vi "Main Page.vi"(8 "error in (no error)":errorcluster, 11 "Node Ptr":T1 format="%.0x") -> (0 "error out":errorcluster)   [LabVIEW 2013, in "PWM System Explorer.lvlib"]
uses:
  PWM System Explorer.lvlib
  <vilib>/NI Veristand/Custom Device API/Custom Device Item Ref.ctl
  NationalInstruments.VeriStand.SystemStorage
  Shared/Constants.vi
  <vilib>/NI Veristand/Custom Device API/Get Item Property (Variant).vi
  <vilib>/NI Veristand/Custom Device API/Set Item Property (Variant).vi
  <vilib>/NI Veristand/Custom Device API/Set Item Property (Double).vi
  <vilib>/NI Veristand/Custom Device Tools/Custom Device Utility Library/NI VeriStand - Search for Item by Name.vi
  <vilib>/NI Veristand/Custom Device API/Custom Device API.lvlib
  <vilib>/NI Veristand/Custom Device Tools/Custom Device Utility Library/Custom Device Utility Library.lvlib
  Shared/PWM Shared.lvlib
panel:
  in  "Remove":bool
  in  "Add":bool
  in  "PWM channels in bitfile":i32[](listbox)=[3]
  in  "Header":cluster{"Section Name":string}={"Section Name"="Custom Device Item Settings"}
  in  "Description":string
  in  "Name":string
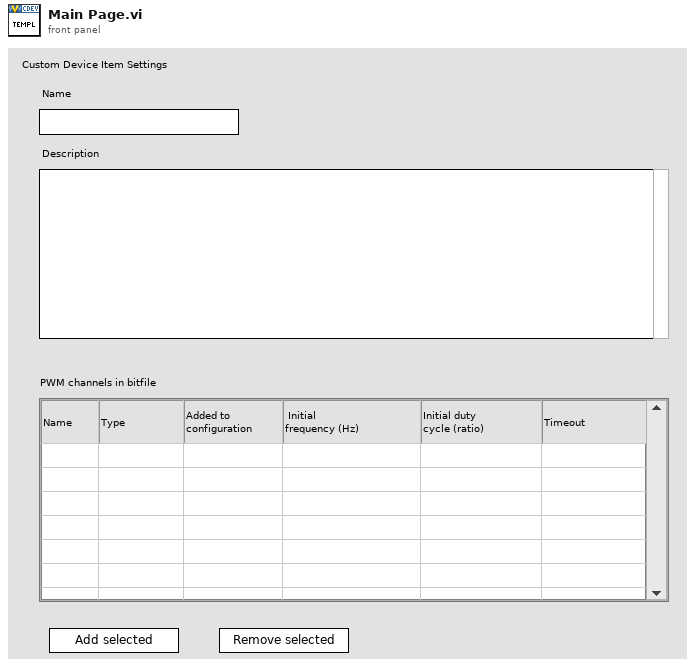
[diagram p1: front panel]
types:
  T1 = typedef "Custom Device API.lvlib/Custom Device Item Ref.ctl" = u64
  T2 = typedef "Custom Device API.lvlib/Custom Device Item Info.ctl" = cluster{"Name":string, "Is Channel":bool, "GUID":string, "Is Waveform":bool}
  T3 = typedef "Custom Device API.lvlib/Custom Device Commands.ctl" = enum16{"Default", "Item renamed", "Shutdown", "Dynamic button pressed"}
  T4 = typedef "Custom Device API.lvlib/Custom Device Pointer.ctl" = refnum<k24>
  T5 = typedef "LVPoint32TypeDef.ctl" = cluster{"Horizontal":i32, "Vertical":i32}
  T6 = typedef "LVRowAndColumnTypeDef.ctl" = cluster{"Row":i32, "Column":i32}
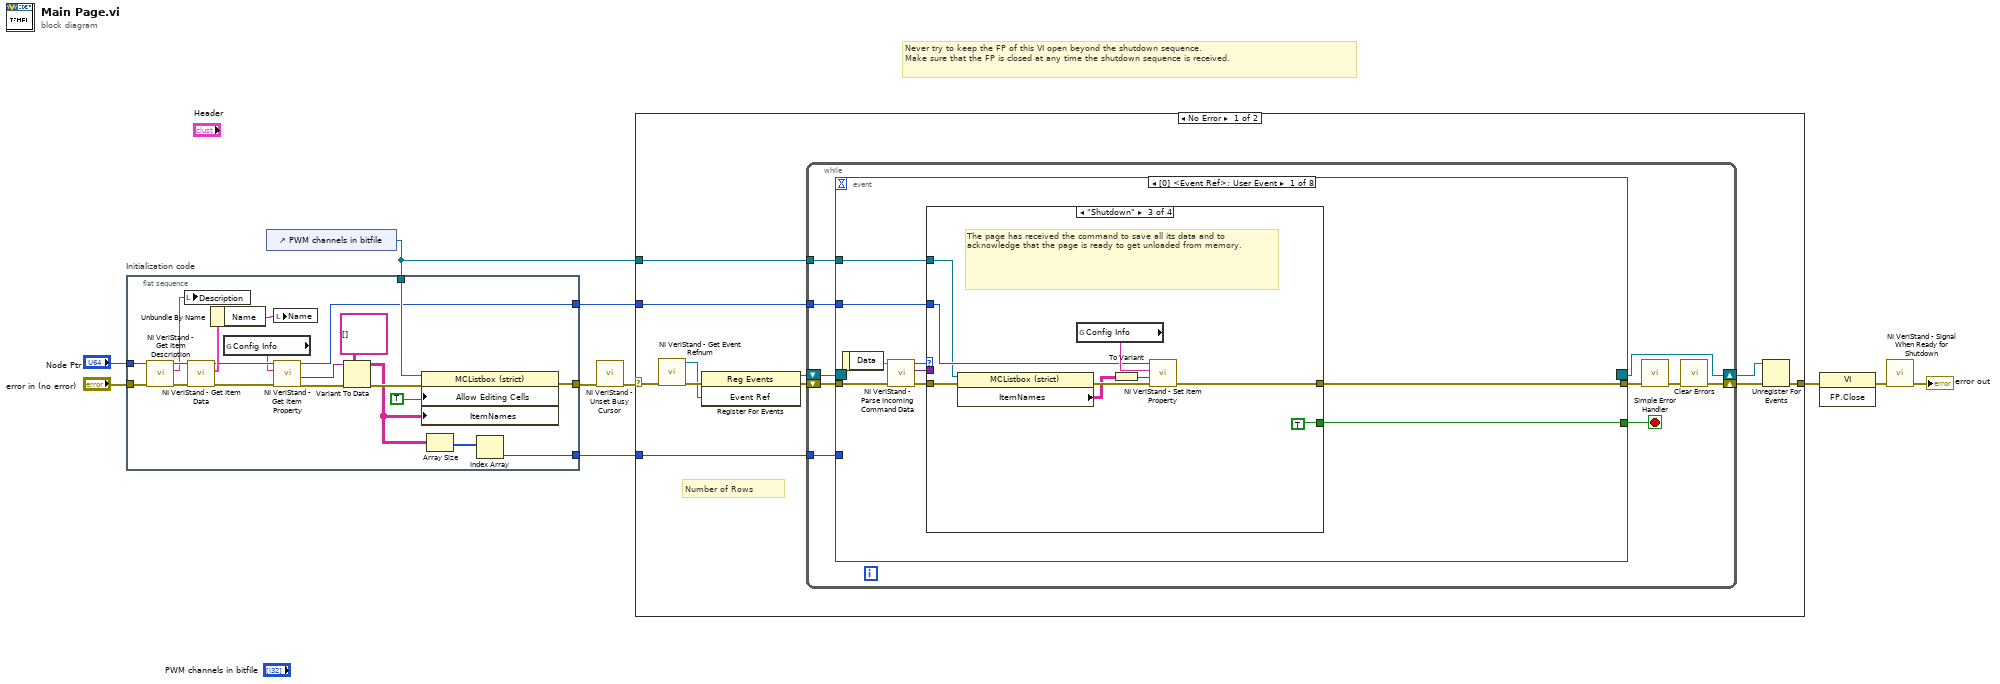
[diagram p0: block diagram]
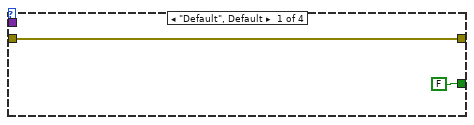
[diagram p2: hidden frame]
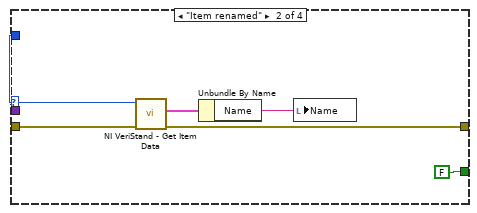
[diagram p3: hidden frame]
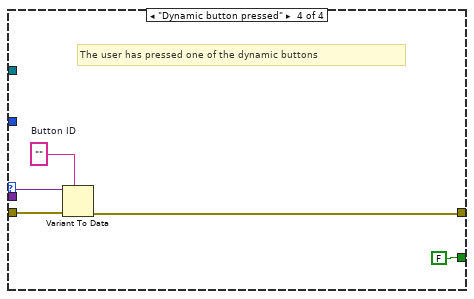
[diagram p4: hidden frame]
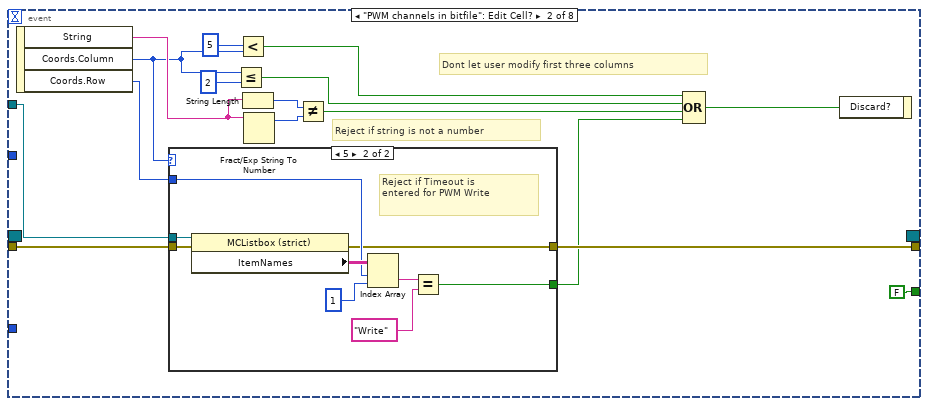
[diagram p5: hidden frame]
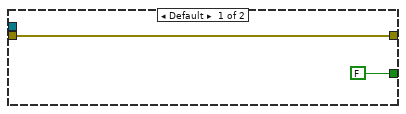
[diagram p6: hidden frame]
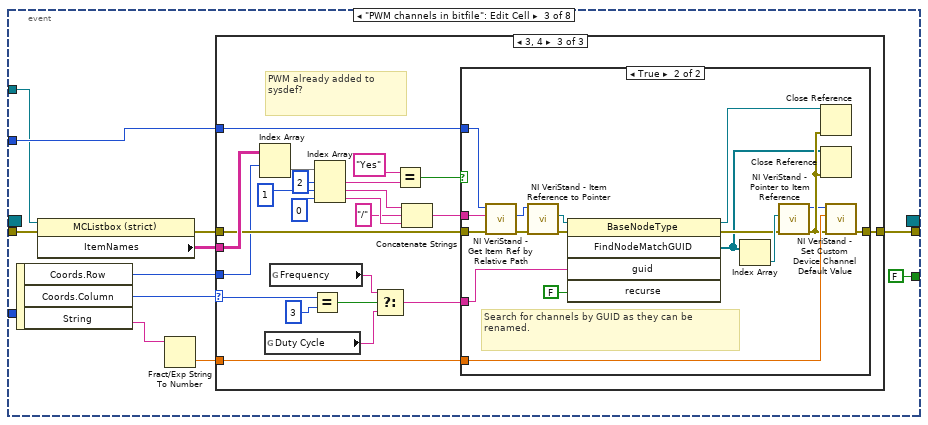
[diagram p7: hidden frame]
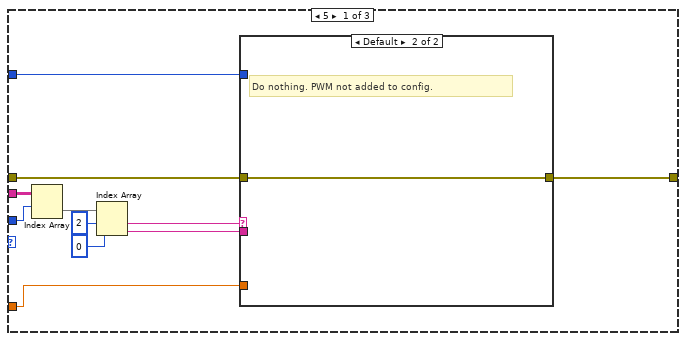
[diagram p8: hidden frame]
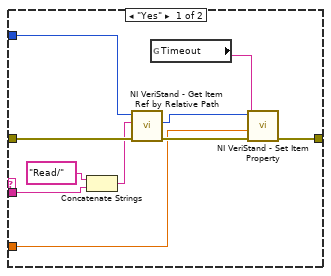
[diagram p9: hidden frame]
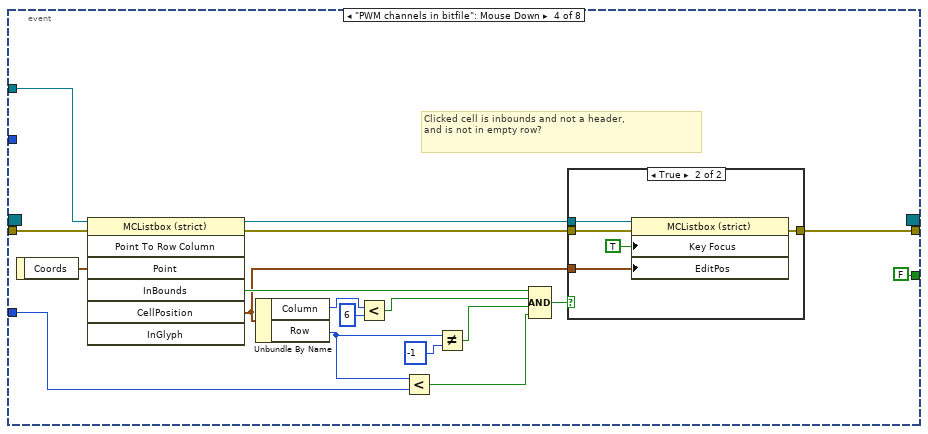
[diagram p12: hidden frame]
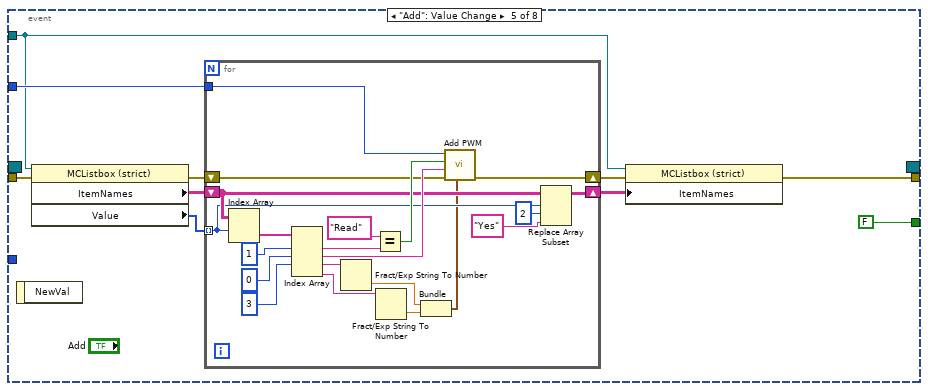
[diagram p14: hidden frame]
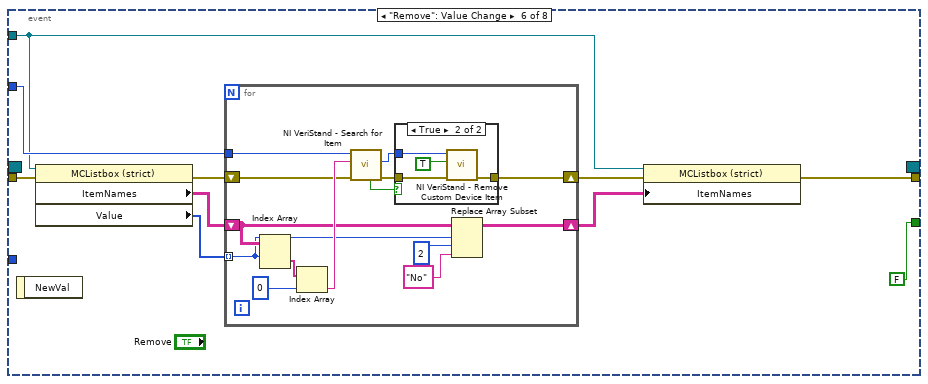
[diagram p15: hidden frame]
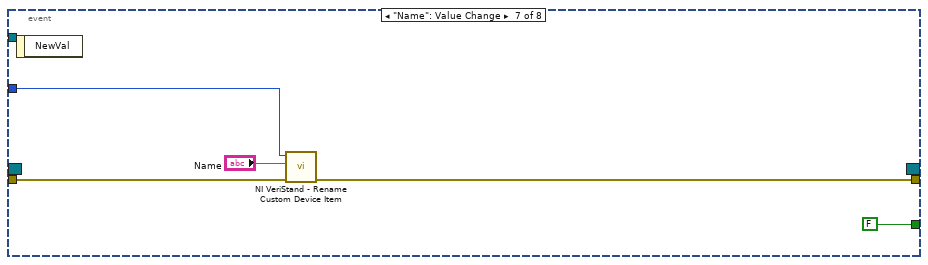
[diagram p17: hidden frame]
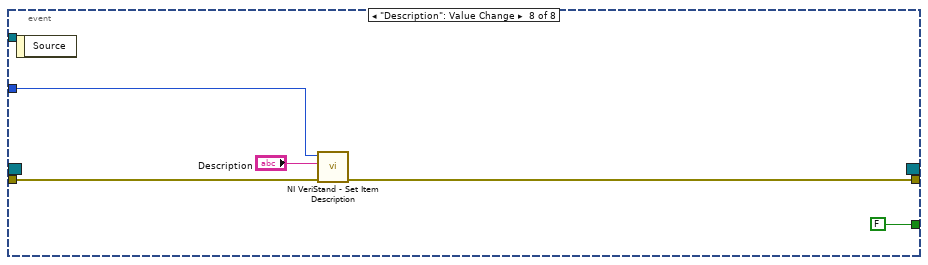
[diagram p18: hidden frame]
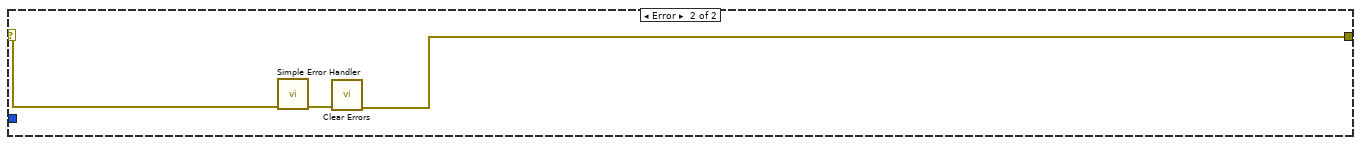
[diagram p19: hidden frame]
diagram:
  # "Never try to keep the FP of this VI open beyond the shutdown sequence.\nMake sure that the FP is closed at any time the shutdown sequence is received."
  n1 = flat-sequence "Initialization code" {
    tunnel: "error in (no error)" -> [w30]
    tunnel: "Node Ptr" -> [w29]
    tunnel: [w23] -> w6
    tunnel: [w17] -> w3
    tunnel: w2 -> [w24]
    tunnel: [w20] -> w1
    frame #0 {
      n2 = call <vilib>:"NI VeriStand - Get Item Description.vi"("error in (no error)"=w30, "Item Ref in"=w29) -> ("error out"=w27:errorcluster, "Description"=w28:string, "Item Ref out"=w31:T1)  [unwired: 7 out]
      n3 = local write "Description"(w28) -> ()
      n4 = call <vilib>:"NI VeriStand - Get Item Data.vi"("error in (no error)"=w27, "Item Ref in"=w31) -> ("error out"=w18:errorcluster, "Item Info"=w26:T2, "Item Ref out"=w19:T1)  [unwired: 7 out]
      n5 = Unbundle By Name(w26) -> ("Name"=w25:string)
      n6 = global read "Constants.vi" "Config Info"() -> (w11:string)
      n7 = local write "Name"(w25) -> ()
      n8 = call-poly <vilib>:"NI VeriStand - Get Item Property.vi"("error in (no error)"=w18, "Property Name"=w11, "Item Ref in"=w19) -> ("error out"=w14:errorcluster, "Value"=w15:variant, "Item Ref out"=w17:T1)  [unwired: 5 in, 1 out]
      n9 = Variant To Data(error in=w14, type=string[][] [] ("Item Names"), Variant=w15) -> (data=w12:string[][], error out=w13:errorcluster)
      n10 = property class="MCListbox (strict)"(reference=w24, error in=w13, "Allow Editing Cells"=TRUE, "ItemNames"=w12) -> (error out=w23:errorcluster)  [unwired: 1 out]
      n11 = Array Size(array=w12) -> (size(s)=w21:i32[])
      n12 = Index Array(array=w21) -> (element=w20:i32)  [unwired: 1 in]
    }
  }
  n13 = control-ref of="PWM channels in bitfile"() -> (w2:refnum<vi>)
  n14 = call <vilib>:"NI VeriStand - Unset Busy Cursor.vi"("error in (no error)"=w6) -> ("error out"=w5:errorcluster)  [unwired: 10 out]
  n15 = case shown="No Error" w5 {
    selector: w5 -> [w35 w282]
    tunnel: [w39 w280] -> w10
    tunnel: w3 -> [w34 _]
    tunnel: w2 -> [w33 _]
    tunnel: w1 -> [w32 _]
    frame No Error {
      # "Number of Rows"
      n16 = call <vilib>:"NI VeriStand - Get Event Refnum.vi"("error in (no error)"=w35) -> ("error out"=w42:errorcluster, "Event Ref"=w38:refnum<user-event>)  [unwired: 9 out]
      n17 = register-events(error in=w42, w38) -> (reference out=w36:refnum<event-registration>, error out=w37:errorcluster)  [unwired: 1 in]
      n18 = while {
        tunnel: w34 -> [w48]
        shift-right: [w45] -> w40
        shift-left: w37 -> [w51]
        shift-right: [w52] -> w41
        shift-left: w36 -> [w50]
        tunnel: w33 -> [w44]
        tunnel: w32 -> [w43]
        stop <- w49 stop-if-true
        n19 = event shown="[0] <Event Ref>: User Event" {
          selector: w50 -> [_ _ _ _ _ _ _ _]
          dyn-events: [_ _ _ _ _ _ _ _] -> w52
          timeout: _ -> [_ _ _ _ _ _ _ _]
          tunnel: w51 -> [w61 w89 w117 w203 w218 w250 w274 w278]
          tunnel: [w57 FALSE FALSE FALSE FALSE FALSE FALSE FALSE] -> w49
          tunnel: [w56 w87 w119 w191 w211 w241 w273 w277] -> w47
          tunnel: w48 -> [w55 _ w120 _ w214 w247 w272 w279]
          tunnel: w44 -> [w53 w90 w118 w189 w212 w243 _ _]
          tunnel: w43 -> [_ _ _ w194 _ _ _ _]
          event User Event {
            n20 = event-data() -> ("Data"=w60:string)  [unwired: 1 out]
            n21 = call <vilib>:"NI VeriStand - Parse Incoming Command Data.vi"("error in (no error)"=w61, "Incoming data"=w60) -> ("error out"=w59:errorcluster, "Outgoing data"=w54:variant, "Action"=w58:T3)  [unwired: 7 out]
            n22 = case shown="\"Shutdown\"" w58 {
              tunnel: w59 -> [w63 w69 w76 w83]
              tunnel: [FALSE FALSE TRUE FALSE] -> w57
              tunnel: [w63 w66 w74 w80] -> w56
              tunnel: w55 -> [_ w68 w72 _]
              tunnel: w54 -> [_ _ _ w82]
              tunnel: w53 -> [_ _ w70 _]
              frame "Default", Default {
              }
              frame "Item renamed" {
                n23 = call <vilib>:"NI VeriStand - Get Item Data.vi"("error in (no error)"=w69, "Item Ref in"=w68) -> ("error out"=w66:errorcluster, "Item Info"=w67:T2)  [unwired: 8 out]
                n24 = Unbundle By Name(w67) -> ("Name"=w65:string)
                n25 = local write "Name"(w65) -> ()
              }
              frame "Shutdown" {
                # "The page has received the command to save all its data and to acknowledge that the page is ready to get unloaded from memory."
                n26 = property class="MCListbox (strict)"(reference=w70, error in=w76) -> (error out=w75:errorcluster, "ItemNames"=w73:string[][])  [unwired: 1 out]
                n27 = global read "Constants.vi" "Config Info"() -> (w77:string)
                n28 = To Variant(anything=w73) -> (Variant=w71:variant)
                n29 = call-poly <vilib>:"NI VeriStand - Set Item Property.vi"("error in (no error)"=w75, "Value"=w71, "Property Name"=w77, "Item Ref in"=w72) -> ("error out"=w74:errorcluster)  [unwired: 5 in, 2 out]
              }
              frame "Dynamic button pressed" {
                w81 = ""  # Button ID
                # "The user has pressed one of the dynamic buttons"
                n30 = Variant To Data(error in=w83, type=w81, Variant=w82) -> (error out=w80:errorcluster)  [unwired: 1 out]
              }
            }
          }
          event "PWM channels in bitfile": Edit Cell? {
            # "Reject if string is not a number"
            # "Dont let user modify first three columns"
            n31 = event-data() -> ("String"=w98:string, "Coords.Column"=w91:i32, "Coords.Row"=w88:i32)  [unwired: 1 out]
            n32 = case shown="5" w91 {
              tunnel: w90 -> [_ w110]
              tunnel: w89 -> [w100 w109]
              tunnel: w88 -> [_ w107]
              tunnel: [FALSE w103] -> w86
              tunnel: [w100 w102] -> w87
              frame Default {
              }
              frame 5 {
                # "Reject if Timeout is \nentered for PWM Write"
                n33 = property class="MCListbox (strict)"(reference=w110, error in=w109) -> (error out=w102:errorcluster, "ItemNames"=w108:string[][])  [unwired: 1 out]
                n34 = Index Array(array=w108, index (row)=w107, index (col)=1 ("disabled index (col)")) -> (element=w105:string)
                n35 = Equal?(x=w105, y="Write") -> (x = y?=w103:bool)
              }
            }
            n36 = Less Or Equal?(x=w91, y=2) -> (x <= y?=w95:bool)
            n37 = Less?(x=5, y=w91) -> (x < y?=w93:bool)
            n38 = String Length(string=w98) -> (length=w97:i32)
            n39 = Fract/Exp String To Number(string=w98) -> (offset past number=w96:i32)  [unwired: 3 in, 1 out]
            n40 = Not Equal?(x=w97, y=w96) -> (x != y?=w85:bool)
            n41 = Compound Arithmetic op=OR(w93, w95, w85, w86) -> (w84:bool)
            n42 = event-data("Discard?"=w84) -> ()  [unwired: 1 in, 1 out]
          }
          event "PWM channels in bitfile": Edit Cell {
            n43 = event-data() -> ("Coords.Row"=w113:i32, "Coords.Column"=w114:i32, "String"=w112:string)  [unwired: 1 out]
            n44 = property class="MCListbox (strict)"(reference=w118, error in=w117) -> (error out=w116:errorcluster, "ItemNames"=w121:string[][])  [unwired: 1 out]
            n45 = Fract/Exp String To Number(string=w112) -> (number=w111:dbl)  [unwired: 3 in, 1 out]
            n46 = case shown="3, 4" w114 {
              selector: w114 -> [_ _ w147]
              tunnel: w121 -> [w132 _ w167]
              tunnel: w120 -> [w123 _ w153]
              tunnel: [w124 w144 w152] -> w119
              tunnel: w111 -> [w122 _ w151]
              tunnel: w116 -> [w131 w144 w150]
              tunnel: w113 -> [w130 _ w146]
              frame 5 {
                n47 = Index Array(array=w132, index (row)=w130) -> (element=w129:string[])  [unwired: 1 in]
                n48 = Index Array(array=w129, index #1=2 ("index"), index #2=0 ("index")) -> (element #1=w127:string, element #2=w125:string)
                n49 = case shown="Default" w127 {
                  tunnel: w131 -> [w140 w143]
                  tunnel: w125 -> [w141 _]
                  tunnel: [w137 w143] -> w124
                  tunnel: w123 -> [w139 _]
                  tunnel: w122 -> [w135 _]
                  frame "Yes" {
                    n50 = Concatenate Strings("Read/" ("string"), w141) -> (w136:string)
                    n51 = call <vilib>:"NI VeriStand - Get Item Ref by Relative Path.vi"("error in"=w140, "Relative Item Path"=w136, "Section Ref in"=w139) -> ("error out"=w138:errorcluster, "Item Ref"=w133:T1)  [unwired: 5 in, 2 out]
                    n52 = global read "Constants.vi" "Timeout"() -> (w134:string)
                    n53 = call-poly <vilib>:"NI VeriStand - Set Item Property.vi"("error in (no error)"=w138, "Value"=w135, "Property Name"=w134, "Item Ref in"=w133) -> ("error out"=w137:errorcluster)  [unwired: 5 in, 2 out]
                  }
                  frame Default {
                    # "Do nothing. PWM not added to config."
                  }
                }
              }
              frame Default {
                # "This should have been filtered out in Edit Cell? case. Dont throw an error. Any edits that happen should be cosmetic only"
              }
              frame 3, 4 {
                # "PWM already added to sysdef?"
                n54 = Index Array(array=w167, index (row)=w146) -> (element=w166:string[])  [unwired: 1 in]
                n55 = global read "Constants.vi" "Duty Cycle"() -> (w149:string)
                n56 = global read "Constants.vi" "Frequency"() -> (w148:string)
                n57 = Equal?(x=w147, y=3) -> (x = y?=w160:bool)
                n58 = Index Array(array=w166, index #1=2 ("index"), index #2=1 ("index"), index #3=0 ("index")) -> (element #1=w164:string, element #2=w159:string, element #3=w158:string)
                n59 = Select(t=w148, s=w160, f=w149) -> (s? t:f=w145:string)
                n60 = Equal?(x="Yes", y=w164) -> (x = y?=w162:bool)
                n61 = Concatenate Strings(w159, "/" ("string"), w158) -> (w154:string)
                n62 = case shown="True" w162 {
                  tunnel: w151 -> [_ w181]
                  tunnel: w154 -> [_ w184]
                  tunnel: w153 -> [_ w185]
                  tunnel: [w168 w183] -> w152
                  tunnel: w150 -> [w168 w182]
                  tunnel: w145 -> [_ w171]
                  frame False {
                    # "PWM not added to\nsysdef. Move on."
                  }
                  frame True {
                    # "Search for channels by GUID as they can be renamed."
                    n63 = call <vilib>:"NI VeriStand - Get Item Ref by Relative Path.vi"("error in"=w182, "Relative Item Path"=w184, "Section Ref in"=w185) -> ("error out"=w177:errorcluster, "Item Ref"=w170:T1)  [unwired: 5 in, 2 out]
                    n64 = call <vilib>:"NI VeriStand - Item Reference to Pointer.vi"("error in (no error)"=w177, "Item Ref in"=w170) -> ("error out"=w180:errorcluster, "Node Pointer"=w179:T4)  [unwired: 6 in, 2 out]
                    n65 = invoke class="BaseNodeType" method="FindNodeMatchGUID"(reference=w179, error in=w180, "guid"=w171, "recurse"=FALSE) -> (reference out=w172:T4, error out=w175:errorcluster, "FindNodeMatchGUID"=w173:refnum<k24>[])  [unwired: 1 in, 2 out]
                    n66 = Index Array(array=w173) -> (element=w176:refnum<k24>)  [unwired: 1 in]
                    n67 = call <vilib>:"NI VeriStand - Pointer to Item Reference.vi"("error in (no error)"=w175, "Node Pointer"=w176) -> ("error out"=w174:errorcluster, "Item Ref out"=w169:T1)  [unwired: 8 in]
                    n68 = Close Reference(reference=w172, error in (no error)=w174) -> ()  [unwired: 1 out]
                    n69 = Close Reference(reference=w173, error in (no error)=w174) -> ()  [unwired: 1 out]
                    n70 = call <vilib>:"NI VeriStand - Set Custom Device Channel Default Value.vi"("error in (no error)"=w174, "Default Value"=w181, "Channel Ref in"=w169) -> ("error out"=w183:errorcluster)  [unwired: 7 in, 1 out]
                  }
                }
              }
            }
          }
          event "PWM channels in bitfile": Mouse Down {
            # "Clicked cell is inbounds and not a header,\nand is not in empty row?"
            n71 = event-data() -> ("Coords"=w202:T5)  [unwired: 1 out]
            n72 = invoke class="MCListbox (strict)" method="Point To Row Column"(reference=w189, error in=w203, "Point"=w202) -> (reference out=w198:refnum<vi>, error out=w197:errorcluster, "InBounds"=w199:bool, "CellPosition"=w195:T6)  [unwired: 4 in, 3 out]
            n73 = Unbundle By Name(w195) -> ("Column"=w188:i32, "Row"=w193:i32)
            n74 = Less?(x=w188, y=6) -> (x < y?=w186:bool)
            n75 = Less?(x=w193, y=w194) -> (x < y?=w192:bool)
            n76 = Not Equal?(x=w193, y=-1) -> (x != y?=w201:bool)
            n77 = Compound Arithmetic op=AND(w199, w186, w201, w192) -> (w196:bool)
            n78 = case shown="True" w196 {
              tunnel: w195 -> [_ w209]
              tunnel: w198 -> [_ w207]
              tunnel: w197 -> [w204 w206]
              tunnel: [w204 w205] -> w191
              frame False {
              }
              frame True {
                n79 = property on="Property Node" class="MCListbox (strict)"(reference=w207, error in=w206, "Key Focus"=TRUE, "EditPos"=w209) -> (error out=w205:errorcluster)  [unwired: 1 out]
              }
            }
          }
          event "Add": Value Change {
            n80 = event-data() -> ()  [unwired: 2 out]
            n81 = property class="MCListbox (strict)"(reference=w212, error in=w218) -> (error out=w215:errorcluster, "ItemNames"=w216:string[][], "Value"=w217:i32[])  [unwired: 1 out]
            n82 = for {
              tunnel: w217 -> [w225] mode=indexing
              shift-right: [w240] -> w213
              shift-left: w215 -> [w228]
              tunnel: w214 -> [w229]
              shift-right: [w227] -> w210
              shift-left: w216 -> [w226]
              n83 = Index Array(array=w226, index (row)=w225) -> (element=w239:string[])  [unwired: 1 in]
              n84 = Index Array(array=w239, index #1=1 ("index"), index #2=0 ("index"), index #3=3 ("index")) -> (element #1=w237:string, element #2=w234:string, element #3=w232:string, element #4=w230:string)  [unwired: 1 in]
              n85 = Fract/Exp String To Number(string=w232) -> (number=w222:dbl)  [unwired: 3 in, 1 out]
              n86 = Equal?(x="Read", y=w237) -> (x = y?=w235:bool)
              n87 = Fract/Exp String To Number(string=w230) -> (number=w221:dbl)  [unwired: 3 in, 1 out]
              n88 = Bundle(w222, w221) -> (w220:cluster{dbl, dbl})  [unwired: 1 in]
              n89 = call "Add PWM.vi"("PWM Properties"=w220, "error in(no error)"=w228, "PWM Name"=w234, "Read?"=w235, "CD Ref in"=w229) -> ("error out"=w240:errorcluster)  [unwired: 5 in, 1 out]
              n90 = Replace Array Subset(array=w226, new element="Yes" ("new element/subarray"), index (row)=w225, index (col)=2 ("disabled index (col)")) -> (w227:string[][])
            }
            n91 = property class="MCListbox (strict)"(reference=w212, error in=w213, "ItemNames"=w210) -> (error out=w211:errorcluster)  [unwired: 1 out]
          }
          event "Remove": Value Change {
            n92 = event-data() -> ()  [unwired: 2 out]
            n93 = property class="MCListbox (strict)"(reference=w243, error in=w250) -> (error out=w246:errorcluster, "ItemNames"=w248:string[][], "Value"=w249:i32[])  [unwired: 1 out]
            n94 = for {
              tunnel: w249 -> [w254] mode=indexing
              tunnel: w247 -> [w262]
              shift-right: [w258] -> w242
              shift-left: w246 -> [w261]
              shift-right: [w256] -> w244
              shift-left: w248 -> [w255]
              n95 = Index Array(array=w255, index (row)=w254) -> (element=w253:string[])  [unwired: 1 in]
              n96 = Index Array(array=w253, index=0) -> (element=w263:string)
              n97 = call-poly <vilib>:"NI VeriStand - Search for Item.vi"("error in"=w261, "Item Name"=w263, "Section Ref in"=w262) -> ("error out"=w260:errorcluster, "Item Ref"=w259:T1, "Found"=w257:bool)  [unwired: 5 in, 1 out]
              n98 = case shown="True" w257 {
                tunnel: w260 -> [w265 w269]
                tunnel: w259 -> [_ w268]
                tunnel: [w265 w266] -> w258
                frame False {
                }
                frame True {
                  n99 = call <vilib>:"NI VeriStand - Remove Custom Device Item.vi"("error in (no error)"=w269, "Force Delete (F)"=TRUE, "Item Ref in"=w268) -> ("error out"=w266:errorcluster)  [unwired: 7 in, 1 out]
                }
              }
              n100 = Replace Array Subset(array=w255, new element="No" ("element"), index (row)=w254, index (col)=2 ("index")) -> (w256:string[][])
            }
            n101 = property class="MCListbox (strict)"(reference=w243, error in=w242, "ItemNames"=w244) -> (error out=w241:errorcluster)  [unwired: 1 out]
          }
          event "Name": Value Change {
            n102 = event-data() -> ()  [unwired: 2 out]
            n103 = call <vilib>:"NI VeriStand - Rename Custom Device Item.vi"("error in (no error)"=w274, "New Name"="Name", "Item Ref in"=w272) -> ("error out"=w273:errorcluster)  [unwired: 1 in, 7 out]
          }
          event "Description": Value Change {
            n104 = event-data() -> ()  [unwired: 2 out]
            n105 = call <vilib>:"NI VeriStand - Set Item Description.vi"("error in (no error)"=w278, "Description"="Description", "Item Ref in"=w279) -> ("error out"=w277:errorcluster)  [unwired: 8 out]
          }
        }
        n106 = call <vilib>:"Simple Error Handler.vi"("error in (no error)"=w47) -> ("error out"=w46:errorcluster)  [unwired: 1 in, 7 out]
        n107 = call <vilib>:"Clear Errors.vi"("error in (no error)"=w46) -> ("error out"=w45:errorcluster)  [unwired: 6 out]
      }
      n108 = Unregister For Events(event registration refnum=w41, error in=w40) -> (error out=w39:errorcluster)
    }
    frame Error {
      n109 = call <vilib>:"Simple Error Handler.vi"("error in (no error)"=w282) -> ("error out"=w281:errorcluster)  [unwired: 1 in, 7 out]
      n110 = call <vilib>:"Clear Errors.vi"("error in (no error)"=w281) -> ("error out"=w280:errorcluster)  [unwired: 6 out]
    }
  }
  n111 = invoke class="VI" method="FP.Close"(error in=w10) -> (error out=w9:errorcluster)  [unwired: 2 in, 2 out]
  n112 = call <vilib>:"NI VeriStand - Signal When Ready for Shutdown.vi"("error in (no error)"=w9) -> ("error out"=→"error out":errorcluster)  [unwired: 10 out]
